vi "Create Resources.vi"() -> (4 "config.resources":T1, 6 "sync.resources":T2, 8 "time.resources":T5)   [LabVIEW 2015]
doc: "Creates and initializes resources for the instrument design libraries.\n\n<B>Output Parameters</B>\n\n<B>config.resources</B> contains references to the configuration registers.\n\n<B>sync.resources</B> contains references to the synchronization registers.\n\n<B>time.resources</B> contains references to the time registers."
uses:
  <instrlib>/niUsrpRio/Time/v1/FPGA/Private/Time Resources.ctl
  <instrlib>/niUsrpRio/Time/v1/FPGA/Private/Future Event Resources.ctl
  <instrlib>/niUsrpRio/Synchronization/v1/FPGA/Private/Resources.ctl
  <instrlib>/niUsrpRio/Time/v1/FPGA/niUsrpRio Time v1 FPGA.lvlib
  <instrlib>/niUsrpRio/Config/v1/FPGA/niUsrpRio Config v1 FPGA.lvlib
  <instrlib>/niUsrpRio/Synchronization/v1/FPGA/niUsrpRio Synchronization v1 FPGA.lvlib
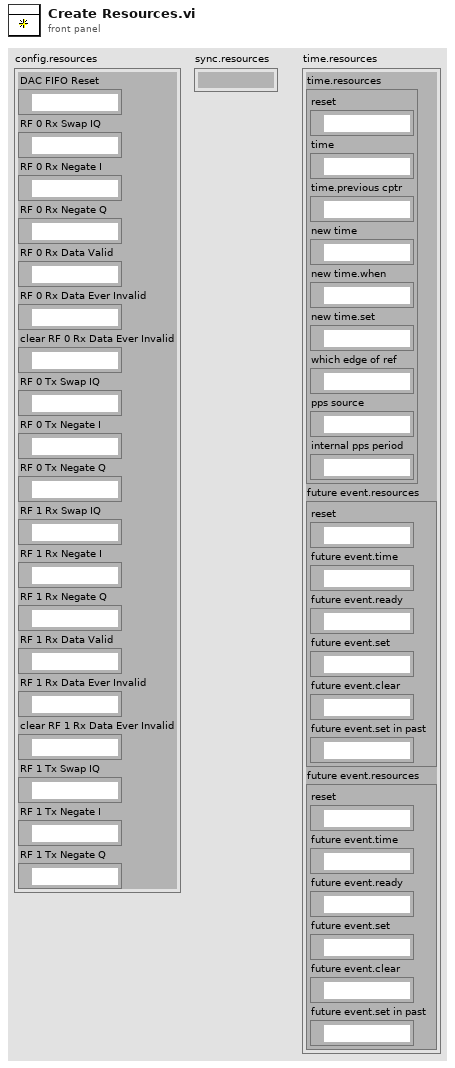
[diagram p1: front panel]
types:
  T1 = cluster{"DAC FIFO Reset":refnum<k21>, "RF 0 Rx Swap IQ":refnum<k21>, "RF 0 Rx Negate I":refnum<k21>, "RF 0 Rx Negate Q":refnum<k21>, "RF 0 Rx Data Valid":refnum<k21>, "RF 0 Rx Data Ever Invalid":refnum<k21>, "clear RF 0 Rx Data Ever Invalid":refnum<k21>, "RF 0 Tx Swap IQ":refnum<k21>, "RF 0 Tx Negate I":refnum<k21>, "RF 0 Tx Negate Q":refnum<k21>, "RF 1 Rx Swap IQ":refnum<k21>, "RF 1 Rx Negate I":refnum<k21>, "RF 1 Rx Negate Q":refnum<k21>, "RF 1 Rx Data Valid":refnum<k21>, "RF 1 Rx Data Ever Invalid":refnum<k21>, "clear RF 1 Rx Data Ever Invalid":refnum<k21>, "RF 1 Tx Swap IQ":refnum<k21>, "RF 1 Tx Negate I":refnum<k21>, "RF 1 Tx Negate Q":refnum<k21>}
  T2 = typedef "niUsrpRio Synchronization v1 FPGA.lvlib/Resources.ctl" = cluster{"master":refnum<k21>, "meas.enable":refnum<k21>, "meas.ready":refnum<k21>, "meas.reset":refnum<k21>, "meas.arm":refnum<k21>, "meas.valid":refnum<k21>, "meas.value":refnum<k21>, "meas.oversample factor":refnum<k21>, "cptr":refnum<k21>, "cptr.adjust":refnum<k21>, "cptr.period":refnum<k21>}
  T3 = typedef "niUsrpRio Time v1 FPGA.lvlib/Time Resources.ctl" = cluster{"reset":refnum<k21>, "time":refnum<k21>, "time.previous cptr":refnum<k21>, "new time":refnum<k21>, "new time.when":refnum<k21>, "new time.set":refnum<k21>, "which edge of ref":refnum<k21>, "pps source":refnum<k21>, "internal pps period":refnum<k21>}
  T4 = typedef "niUsrpRio Time v1 FPGA.lvlib/Future Event Resources.ctl" = cluster{"reset":refnum<k21>, "future event.time":refnum<k21>, "future event.ready":refnum<k21>, "future event.set":refnum<k21>, "future event.clear":refnum<k21>, "future event.set in past":refnum<k21>}
  T5 = cluster{"time.resources":T3, "future event.resources":T4, "future event.resources":T4}
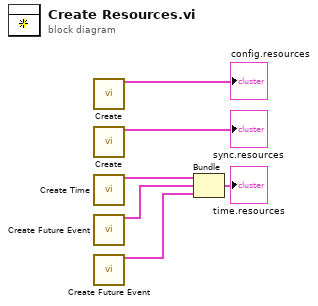
[diagram p0: block diagram]
diagram:
  n1 = call <instrlib>:"Create.vi"() -> ("resources"=→"config.resources":T1)  [unwired: 15 in]
  n2 = call <instrlib>:"Create.vi"() -> ("sync.resources"=→"sync.resources":T2)  [unwired: 15 in]
  n3 = call <instrlib>:"Create Time.vi"() -> ("time.resources"=w6:T3)  [unwired: 15 in]
  n4 = call <instrlib>:"Create Future Event.vi"() -> ("future event.resources"=w5:T4)  [unwired: 15 in]
  n5 = call <instrlib>:"Create Future Event.vi"() -> ("future event.resources"=w4:T4)  [unwired: 15 in]
  n6 = Bundle("time.resources"=w6, "future event.resources"=w5, "future event.resources"=w4) -> (→"time.resources":T5)  [unwired: 1 in]
